vi "Attenuator_AxisInit.vi"(2 "error in (no error)":errorcluster caption="错误输入（无错误）", 3 "Axis":u16) -> (0 "error out":errorcluster caption="错误输出")   [LabVIEW 2018]
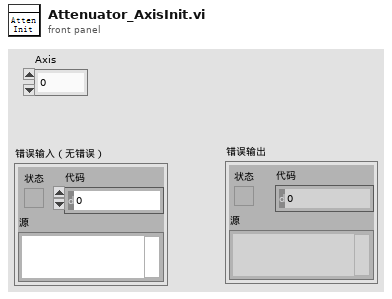
[diagram p1: front panel]
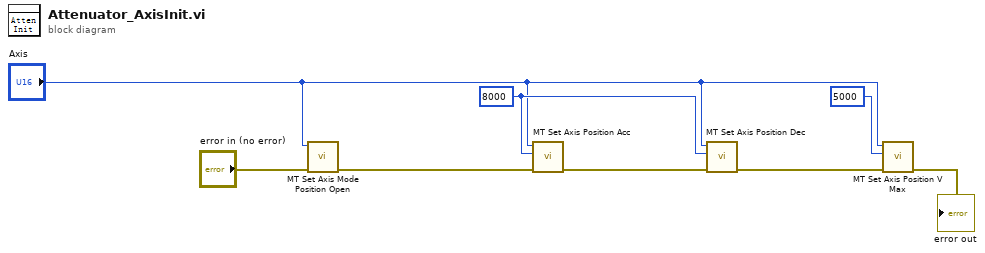
[diagram p0: block diagram]
diagram:
  w8 = 8000 ("Value")
  n1 = call "MT Set Axis Mode Position Open.vi"("error in (no error)"="error in (no error)", "AObj"="Axis") -> ("error out"=w5:errorcluster)  [unwired: 8 in, 1 out]
  n2 = call "MT Set Axis Position Acc.vi"("error in (no error)"=w5, "Value"=w8, "AObj"="Axis") -> ("error out"=w4:errorcluster)  [unwired: 7 in, 1 out]
  n3 = call "MT Set Axis Position Dec.vi"("error in (no error)"=w4, "Value"=w8, "AObj"="Axis") -> ("error out"=w3:errorcluster)  [unwired: 7 in, 1 out]
  n4 = call "MT Set Axis Position V Max.vi"("error in (no error)"=w3, "Value"=5000, "AObj"="Axis") -> ("error out"=→"error out":errorcluster)  [unwired: 7 in, 1 out]
